vi "Find PS3 Controller.vi"(8 "error in (no error)":errorcluster) -> (0 "error out":errorcluster, 3 "Controller Reference Out":refnum<k1>)   [LabVIEW 8.6]
doc: "This VI finds the first DualShock 3 controller identified by the operating system as a Joystick."
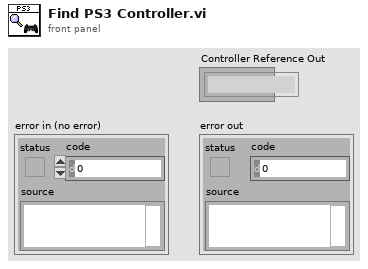
[diagram p1: front panel]
types:
  T1 = cluster{"axes total":u32, "buttons total":u32, "pov total":u32, "device name":string}[]
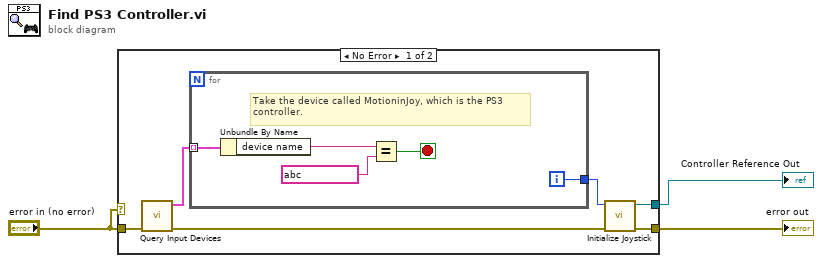
[diagram p0: block diagram]
diagram:
  n1 = case shown="No Error" "error in (no error)" {
    tunnel: "error in (no error)" -> [w9 w15]
    tunnel: [w6 _] -> w3
    tunnel: [w5 w15] -> w2
    frame #0 {
      n2 = call <vilib>:"Query Input Devices.vi"("error in (no error)"=w9) -> ("error out"=w4:errorcluster, "joystick info"=w7:T1)  [unwired: 9 out]
      n3 = for {
        tunnel: w7 -> [w14] mode=indexing
        tunnel: [w10] -> w8
        i -> [w10]
        stop <- w11 stop-if-true
        # "Take the device called MotioninJoy, which is the PS3 controller."
        n4 = Unbundle By Name(w14) -> ("device name"=w13:string)
        n5 = Equal?(x=w13, y=string ?) -> (x = y?=w11:bool)
      }
      n6 = call <vilib>:"Initialize Joystick.vi"("error in (no error)"=w4, "device index"=w8) -> ("error out"=w5:errorcluster, "device ID"=w6:refnum<k1>)  [unwired: 8 out]
    }
    frame #1 {
    }
  }
  "Controller Reference Out" <- w3
  "error out" <- w2
